vi "扭转直到最大.vi"(2 "数组－数值 2":dbl[](array[numeric]), 3 "数组－数值":dbl[](array[numeric])) -> (0 "子数组 2":dbl[](array[numeric]), 1 "子数组":dbl[](array[numeric]))   [LabVIEW 2016]
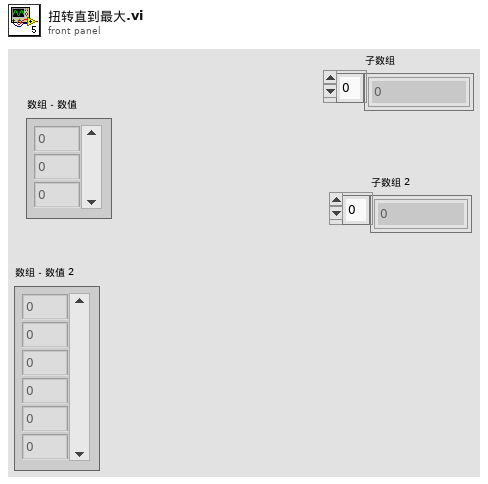
[diagram p1: front panel]
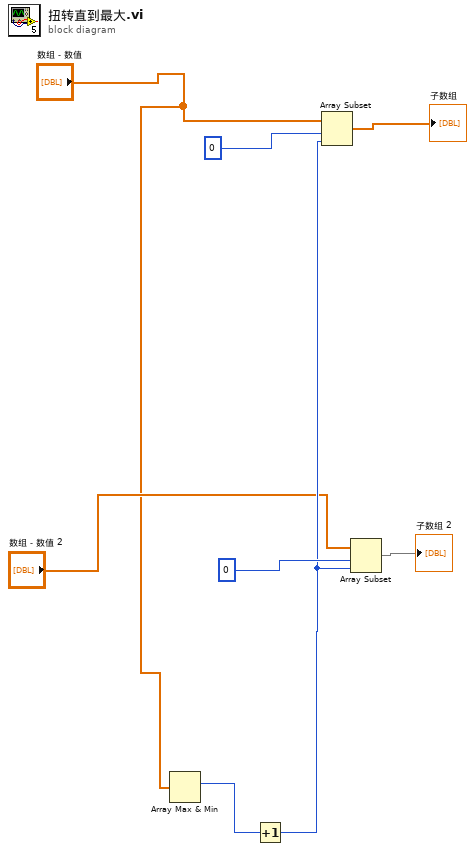
[diagram p0: block diagram]
diagram:
  n1 = Array Max & Min(array="数组－数值") -> (max index (indices)=w3:i32)  [unwired: 3 out]
  n2 = Increment(x=w3) -> (x+1=w6:i32)
  n3 = Array Subset(array="数组－数值", index=0 ("索引"), length=w6) -> (→"子数组":dbl[])
  n4 = Array Subset(array="数组－数值 2", index=0 ("索引"), length=w6) -> (→"子数组 2":dbl[])
